vi "Configure Channel (RTD Normal).vi"(0 "VISA resource name":refnum<visa-resource-name>, 5 "Channel (0001)":string="0001", 7 "Enable Channel (True)":bool=TRUE, 9 "Type and Span":T1={"RTD Type (0 : Pt100)"=0, "Enable Span (False)"=FALSE, "Lower Span (-200.0)"=-200.0, "Upper Span (850.0)"=850.0, "Bias (0)"=0.0} {"Bias (0)" format="%_6g"; "Upper Span (850.0)" min=-99999.0 max=99999.0 step=0.1 format="%.2f"; "Lower Span (-200.0)" min=-99999.0 max=99999.0 step=0.1 format="%.2f"; "RTD Type (0 : Pt100)" items=["Pt100", "Pt100-H", "JPt100", "JPt100-H", "Cu10GE", "Cu10LN", "Cu10WEED", "Cu10BAILEY", "Cu10a392", "Cu10a393", "Cu25", "Cu53", "Cu100", "J263B", "Ni100SAMA", "Ni100DIN", "Ni120", "Pt25", "Pt50", "Pt200WEED", "Cu10G", "Cu50G", "Cu100G", "Pt46G", "Pt100G"]}, 11 "error in (no error)":errorcluster) -> (4 "VISA resource name out":refnum<visa-resource-name>, 6 "Channel":string, 15 "error out":errorcluster)   [LabVIEW 2020, in "Yokogawa GX Series.lvlib"]
doc: "Sets the input range as Resistance Temperature Detector (RTD).\n\nCommand: SRangeAI"
uses:
  <instrlib>/Yokogawa GX Series/Yokogawa GX Series.lvlib
  <instrlib>/Yokogawa GX Series/Private/RTD Range.vi
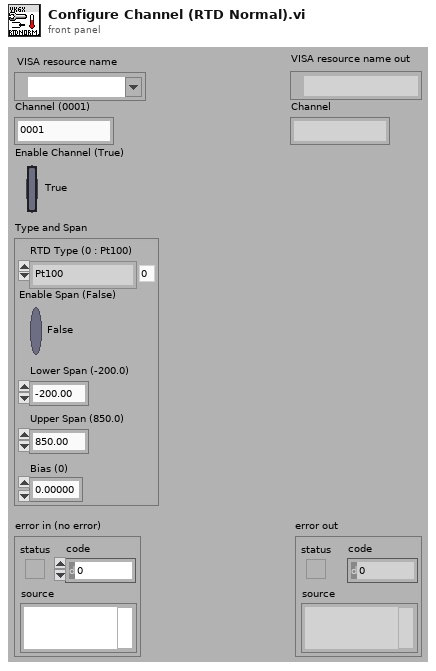
[diagram p1: front panel]
types:
  T1 = cluster{"RTD Type (0 : Pt100)":i32, "Enable Span (False)":bool, "Lower Span (-200.0)":dbl, "Upper Span (850.0)":dbl, "Bias (0)":dbl}
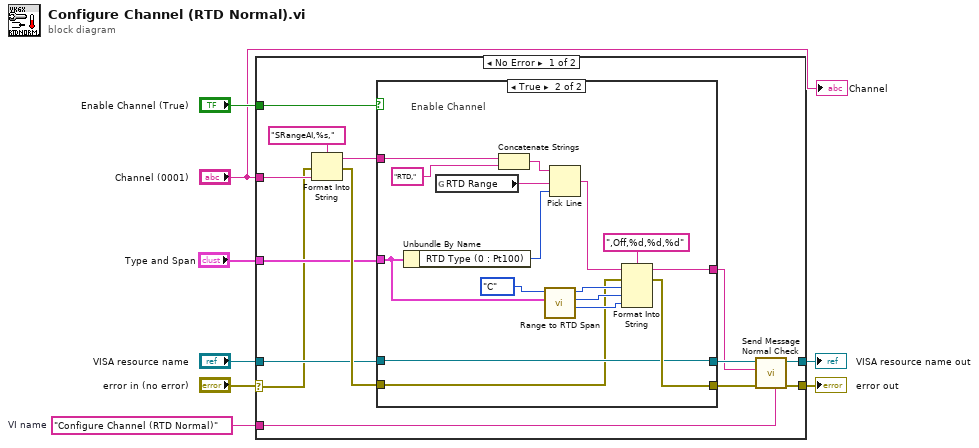
[diagram p0: block diagram]
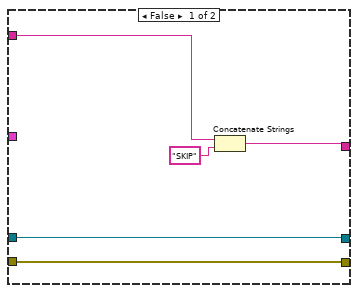
[diagram p2: hidden frame]
diagram:
  w3 = "Configure Channel (RTD Normal)"  # VI name
  n1 = case shown="No Error" "error in (no error)" {
    selector: "error in (no error)" -> [w9 w44]
    tunnel: "Enable Channel (True)" -> [w19 _]
    tunnel: "VISA resource name" -> [w18 w45]
    tunnel: "Type and Span" -> [w17 _]
    tunnel: [w13 w45] -> w5
    tunnel: [w12 w44] -> w4
    tunnel: w3 -> [w11 _]
    tunnel: "Channel (0001)" -> [w10 _]
    frame No Error {
      n2 = Format Into String(format string="SRangeAI,%s,", error in=w9, w10) -> (resulting string=w20:string, error out=w21:errorcluster)  [unwired: 1 in]
      n3 = case shown="True" w19 {
        tunnel: w21 -> [w26 w31]
        tunnel: w20 -> [w27 w42]
        tunnel: [w26 w41] -> w15
        tunnel: w18 -> [w25 w32]
        tunnel: [w25 w32] -> w16
        tunnel: w17 -> [_ w39]
        tunnel: [w23 w36] -> w14
        frame False {
          n4 = Concatenate Strings(w27, "SKIP") -> (w23:string)
        }
        frame True {
          # "Enable Channel"
          n5 = Unbundle By Name(w39) -> ("RTD Type (0 : Pt100)"=w38:i32)
          n6 = global read "RTD Range.vi" "RTD Range"() -> (w28:string)
          n7 = Concatenate Strings(w42, "RTD,") -> (w40:string)
          n8 = call <instrlib>:"Range to RTD Span.vi"("Type and Span"=w39, "Temp. unit (0: C)"=enum16{"C", "F"}."C") -> ("Bias"=w33:i32, "Upper span"=w34:i32, "Lower Span"=w35:i32)  [unwired: 7 in]
          n9 = Pick Line(string ("")=w40, multi-line string=w28, line index=w38) -> (output string=w37:string)
          n10 = Format Into String(format string=",Off,%d,%d,%d", initial string=w37, error in=w31, w35, w34, w33) -> (resulting string=w36:string, error out=w41:errorcluster)
        }
      }
      n11 = call <instrlib>:"Send Message Normal Check.vi"("Source (\"\")"=w11, "error in (no error)"=w15, "Send Message (\"\")"=w14, "VISA resource name"=w16) -> ("error out"=w12:errorcluster, "VISA resource name out"=w13:refnum<visa-resource-name>)  [unwired: 2 in, 4 out]
    }
    frame Error {
    }
  }
  "error out" <- w4
  "VISA resource name out" <- w5
  "Channel" <- "Channel (0001)"
